vi "LChecker.vi"(11 "error in (no error)":errorcluster) -> (3 "DevMode":bool, 4 "Student":bool, 15 "error out":errorcluster)   [LabVIEW 2014, in "Raspberry Pi Compatible Compiler for LabVIEW.lvlib"]
doc: "Checker."
uses:
  Raspberry Pi Compatible Compiler for LabVIEW.lvlib
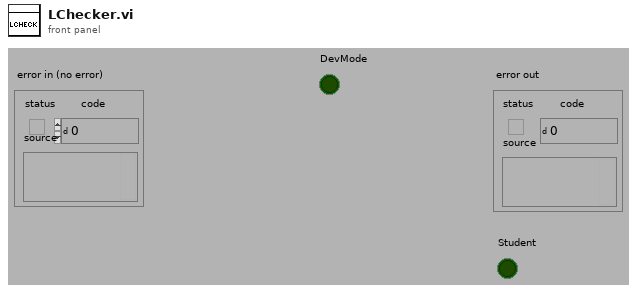
[diagram p1: front panel]
types:
  T1 = enum16{"Invalid", "Expired", "Evaluation", "Activated"}
  T2 = enum32{"invalid app kind", "Development System", "Run Time System", "Student Edition", "Embedded LabVIEW", "Evaluation", "Custom"}
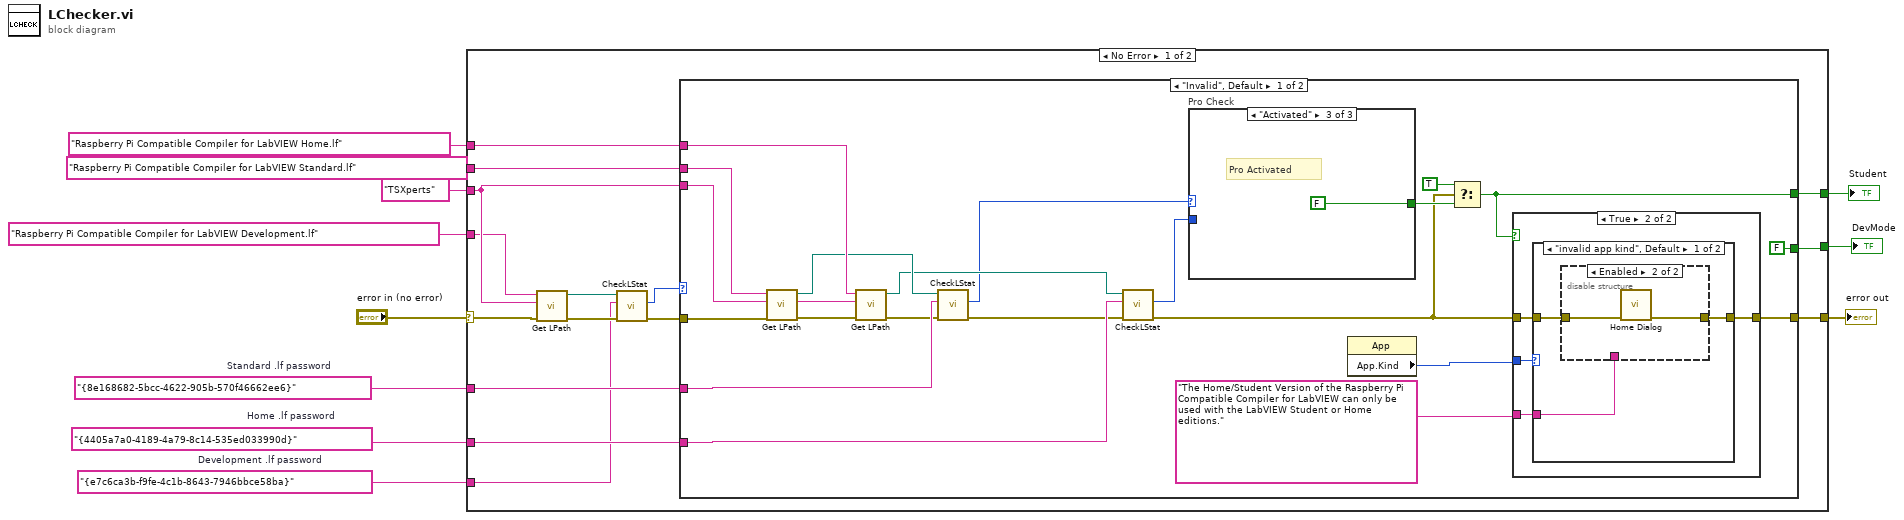
[diagram p0: block diagram]
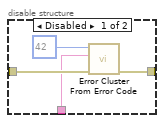
[diagram p3: hidden frame]
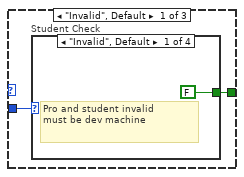
[diagram p5: hidden frame]
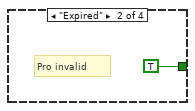
[diagram p6: hidden frame]
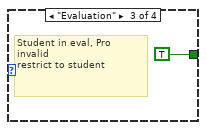
[diagram p7: hidden frame]
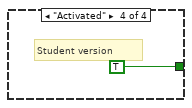
[diagram p8: hidden frame]
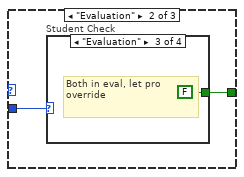
[diagram p9: hidden frame]
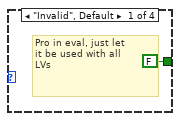
[diagram p10: hidden frame]
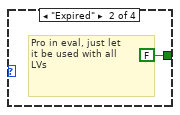
[diagram p11: hidden frame]
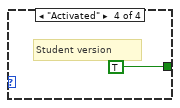
[diagram p12: hidden frame]
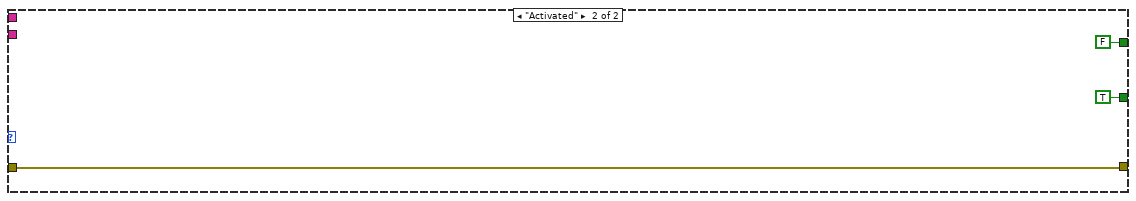
[diagram p13: hidden frame]
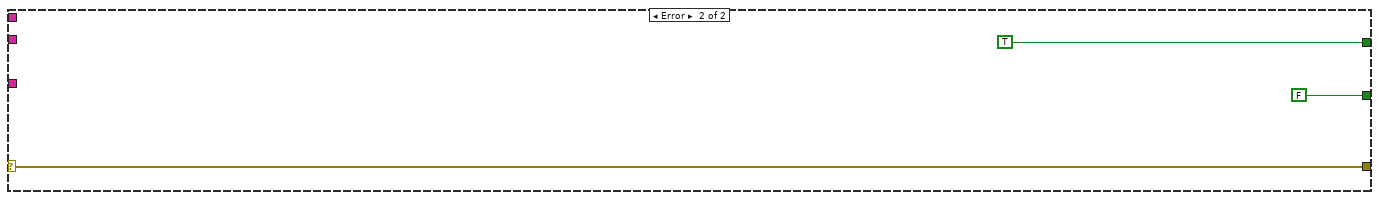
[diagram p14: hidden frame]
diagram:
  w1 = "{e7c6ca3b-f9fe-4c1b-8643-7946bbce58ba}"  # Development .lf password
  w4 = "{4405a7a0-4189-4a79-8c14-535ed033990d}"  # Home .lf password
  w5 = "{8e168682-5bcc-4622-905b-570f46662ee6}"  # Standard .lf password
  n1 = case shown="No Error" "error in (no error)" {
    selector: "error in (no error)" -> [w19 w80]
    tunnel: [w21 w80] -> w10
    tunnel: "Raspberry Pi Compatible Compiler for LabVIEW Standard.lf" ("license file name") -> [w25 _]
    tunnel: "Raspberry Pi Compatible Compiler for LabVIEW Home.lf" ("license file name") -> [w24 _]
    tunnel: "TSXperts" ("company name") -> [w18 _]
    tunnel: w4 -> [w23 _]
    tunnel: [w22 TRUE ("SV")] -> w6
    tunnel: w5 -> [w20 _]
    tunnel: [w16 FALSE ("SV")] -> w3
    tunnel: "Raspberry Pi Compatible Compiler for LabVIEW Development.lf" ("license file name") -> [w17 _]
    tunnel: w1 -> [w13 _]
    frame No Error {
      n2 = call "Get LPath.vi"("error in (no error)"=w19, "company name"=w18, "license file name"=w17) -> ("error out"=w15:errorcluster, "license file path"=w14:path)  [unwired: 7 in]
      n3 = call "CheckLStat.vi"("error in (no error)"=w15, "password"=w13, "license file path"=w14) -> ("license status"=w12:T1)  [unwired: 5 in, 3 out]
      n4 = case shown="\"Invalid\", Default" w12 {
        tunnel: w25 -> [w46 _]
        tunnel: w24 -> [w45 _]
        tunnel: w23 -> [w44 _]
        tunnel: [w43 FALSE ("SV")] -> w22
        tunnel: [w42 w75] -> w21
        tunnel: w20 -> [w41 _]
        tunnel: w18 -> [w40 _]
        tunnel: [FALSE TRUE] -> w16
        tunnel: w15 -> [w38 w75]
        frame "Invalid", Default {
          n5 = call "Get LPath.vi"("error in (no error)"=w38, "company name"=w40, "license file name"=w46) -> ("error out"=w37:errorcluster, "license file path"=w35:path)  [unwired: 7 in]
          n6 = call "Get LPath.vi"("error in (no error)"=w37, "company name"=w40, "license file name"=w45) -> ("error out"=w36:errorcluster, "license file path"=w34:path)  [unwired: 7 in]
          n7 = call "CheckLStat.vi"("error in (no error)"=w36, "password"=w41, "license file path"=w35) -> ("error out"=w26:errorcluster, "license status"=w33:T1)  [unwired: 5 in, 2 out]
          n8 = call "CheckLStat.vi"("error in (no error)"=w26, "password"=w44, "license file path"=w34) -> ("error out"=w28:errorcluster, "license status"=w32:T1)  [unwired: 5 in, 2 out]
          n9 = case "Pro Check" shown="\"Activated\"" w33 {
            tunnel: [w62 w68 FALSE ("SV")] -> w31
            tunnel: w32 -> [w63 w69 _]
            frame "Invalid", Default {
              n10 = case "Student Check" shown="\"Invalid\", Default" w63 {
                tunnel: [FALSE ("SV") TRUE ("SV") TRUE ("SV") TRUE ("SV")] -> w62
                frame "Invalid", Default {
                  # "Pro and student invalid\nmust be dev machine"
                }
                frame "Expired" {
                  # "Pro invalid"
                }
                frame "Evaluation" {
                  # "Student in eval, Pro\ninvalid\nrestrict to student"
                }
                frame "Activated" {
                  # "Student version"
                }
              }
            }
            frame "Evaluation" {
              n11 = case "Student Check" shown="\"Evaluation\"" w69 {
                tunnel: [FALSE ("SV") FALSE ("SV") FALSE ("SV") TRUE ("SV")] -> w68
                frame "Invalid", Default {
                  # "Pro in eval, just let\nit be used with all\nLVs"
                }
                frame "Expired" {
                  # "Pro in eval, just let\nit be used with all\nLVs"
                }
                frame "Evaluation" {
                  # "Both in eval, let pro\noverride"
                }
                frame "Activated" {
                  # "Student version"
                }
              }
            }
            frame "Activated" {
              # "Pro Activated"
            }
          }
          n12 = property class="App"() -> ("App.Kind"=w29:T2)  [unwired: 2 in, 2 out]
          n13 = Select(t=TRUE, s=w28, f=w31) -> (s? t:f=w43:bool)
          n14 = case shown="True" w43 {
            tunnel: w29 -> [_ w51]
            tunnel: w28 -> [w47 w50]
            tunnel: "The Home/Student Version of the Raspberry Pi Compatible Compiler for LabVIEW can only be used with the LabVIEW Student or Home editions." ("password") -> [_ w49]
            tunnel: [w47 w48] -> w42
            frame False {
            }
            frame True {
              n15 = case shown="\"invalid app kind\", Default" w51 {
                tunnel: w50 -> [w54 w61]
                tunnel: w49 -> [w53 _]
                tunnel: [w52 w61] -> w48
                frame "invalid app kind", Default {
                  n16 = disable-structure shown="Enabled" {
                    disable-tunnel: w54 -> [w58 w60]
                    disable-tunnel: w53 -> [w56 _]
                    disable-tunnel: [w55 w59] -> w52
                    frame Disabled {
                      n17 = call <vilib>:"Error Cluster From Error Code.vi"("error in (no error)"=w58, "error message (\"\")"=w56, "error code (0)"=42) -> ("error out"=w55:errorcluster)  [unwired: 6 in]
                    }
                    frame Enabled {
                      n18 = call "Home Dialog.vi"("error in (no error)"=w60) -> ("error out"=w59:errorcluster)  [unwired: 10 in]
                    }
                  }
                }
                frame "Student Edition", "Evaluation" {
                }
              }
            }
          }
        }
        frame "Activated" {
        }
      }
    }
    frame Error {
    }
  }
  "error out" <- w10
  "Student" <- w6
  "DevMode" <- w3
